vi "Add Error Meta.vi"(8 "error in (no error)":errorcluster, 10 "Section Header (Debug Data:)":string="Debug Data:", 11 "Data":variant) -> (0 "error out":errorcluster)   [LabVIEW 2016, in "SLL Debug.lvlib"]
doc: "This VI is useful for adding useful meta data to the error cluster, like the data with which the error occurred.\n\nIf there is no incoming error, no details are added."
uses:
  SLL Debug.lvlib
  <vilib>/addons/_JKI.lib/Serialization/JSON/JKI JSON Serialization.lvlib
panel:
  # "This VI is useful for adding useful meta data to the error cluster, like the data with which the error occurred."
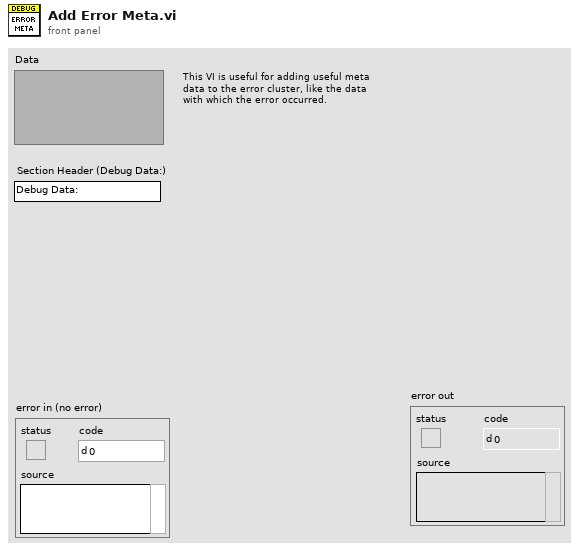
[diagram p1: front panel]
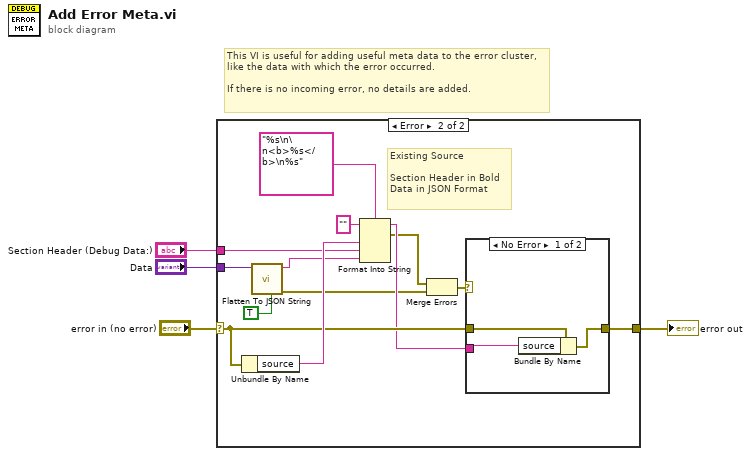
[diagram p0: block diagram]
diagram:
  # "This VI is useful for adding useful meta data to the error cluster, like the data with which the error occurred.\n\nIf there is no incoming error, no details are added."
  n1 = case shown="Error" "error in (no error)" {
    selector: "error in (no error)" -> [w5 w15]
    tunnel: [w5 w14] -> w3
    tunnel: "Section Header (Debug Data:)" -> [_ w12]
    tunnel: "Data" -> [_ w11]
    frame No Error {
    }
    frame Error {
      # "Existing Source\n\nSection Header in Bold\nData in JSON Format"
      n2 = Unbundle By Name(w15) -> ("source"=w17:string)
      n3 = call <vilib>:"Flatten To JSON String.vi"("Enums As String (F)"=TRUE, "Variant"=w11) -> ("error out"=w7:errorcluster, "JSON String"=w9:string)  [unwired: 8 in]
      n4 = Format Into String(format string="%s\n\n<b>%s</b>\n%s", initial string="", w17, w12, w9) -> (resulting string=w13:string, error out=w8:errorcluster)  [unwired: 1 in]
      n5 = Merge Errors(w8, w7) -> (w6:errorcluster)
      n6 = case shown="No Error" w6 {
        tunnel: w15 -> [w21 w22]
        tunnel: [w20 w22] -> w14
        tunnel: w13 -> [w19 _]
        frame No Error {
          n7 = Bundle By Name(cluster=w21, "source"=w19) -> (w20:errorcluster)
        }
        frame Error {
        }
      }
    }
  }
  "error out" <- w3
